vi "Set Default Config.vi"(8 "error in (no error)":errorcluster, 11 "reference in":refnum<k24>) -> (0 "error out":errorcluster, 3 "reference out":refnum<k24>)   [LabVIEW 2019, in "LabNation Scope Driver.lvlib"]
doc: "Configures the Smart Scope with default settings during start up."
uses:
  LabNation Scope Driver.lvlib
  C:/Program Files (x86)/LabNation/SmartScope/DeviceInterface.dll
  Program Files (x86)/LabNation/SmartScope/DeviceInterface.dll
  Typedef/AcquisitionMode.ctl
  Typedef/Coupling.ctl
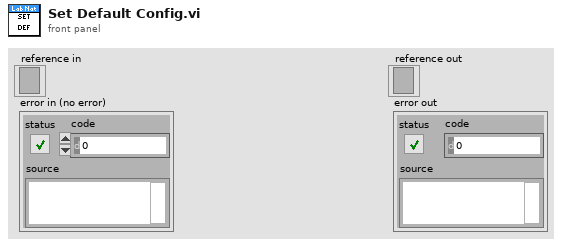
[diagram p1: front panel]
types:
  T1 = typedef "LabNation Scope Driver.lvlib/AcquisitionMode.ctl" = i32
  T2 = typedef "LabNation Scope Driver.lvlib/Coupling.ctl" = i32
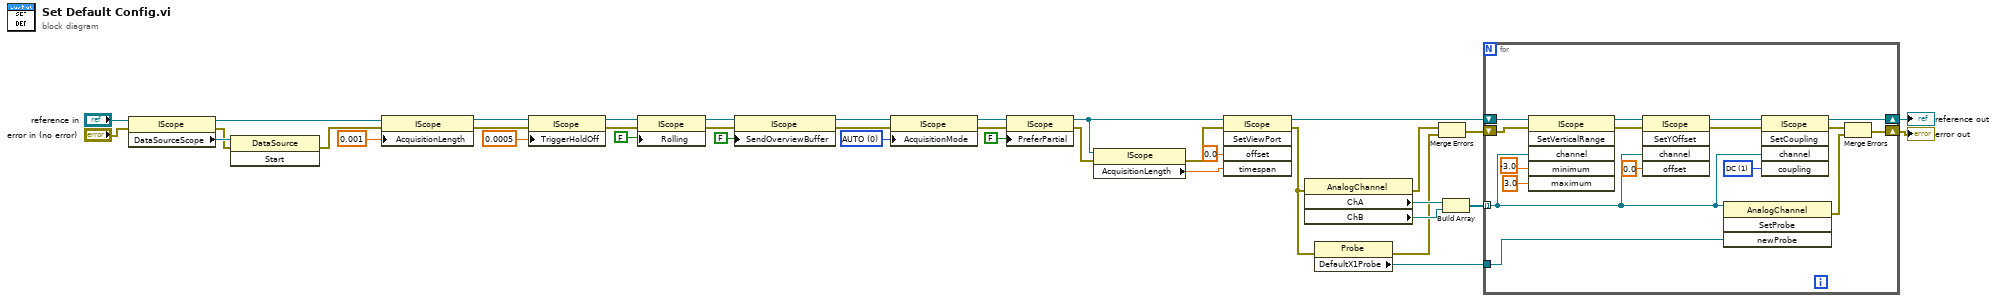
[diagram p0: block diagram]
diagram:
  w32 = T1 0 items=["AUTO", "NORMAL", "SINGLE"] ("AcquisitionMode")
  n1 = property class="IScope"(reference="reference in", error in="error in (no error)") -> (reference out=w38:refnum<k24>, error out=w18:errorcluster, "DataSourceScope"=w29:refnum<k24>)
  n2 = invoke class="DataSource" method="Start"(reference=w29, error in=w18) -> (error out=w37:errorcluster)  [unwired: 1 in, 2 out]
  n3 = property class="IScope"(reference=w38, error in=w37, "AcquisitionLength"=0.001) -> (reference out=w23:refnum<k24>, error out=w17:errorcluster)
  n4 = property class="IScope"(reference=w23, error in=w17, "TriggerHoldOff"=0.0005 ("AcquisitionLength")) -> (reference out=w24:refnum<k24>, error out=w16:errorcluster)
  n5 = property class="IScope"(reference=w24, error in=w16, "Rolling"=FALSE ("LogicAnalyserEnabled")) -> (reference out=w25:refnum<k24>, error out=w15:errorcluster)
  n6 = property class="IScope"(reference=w25, error in=w15, "SendOverviewBuffer"=FALSE) -> (reference out=w26:refnum<k24>, error out=w14:errorcluster)
  n7 = property class="IScope"(reference=w26, error in=w14, "AcquisitionMode"=w32) -> (reference out=w27:refnum<k24>, error out=w13:errorcluster)
  n8 = property class="IScope"(reference=w27, error in=w13, "PreferPartial"=FALSE) -> (reference out=w35:refnum<k24>, error out=w12:errorcluster)
  n9 = property class="IScope"(reference=w35, error in=w12) -> (error out=w11:errorcluster, "AcquisitionLength"=w36:dbl)  [unwired: 1 out]
  n10 = invoke class="IScope" method="SetViewPort"(reference=w35, error in=w11, "offset"=0.0, "timespan"=w36) -> (reference out=w20:refnum<k24>, error out=w7:errorcluster)  [unwired: 1 in, 3 out]
  n11 = property class="AnalogChannel"(error in=w7) -> (error out=w5:errorcluster, "ChA"=w19:refnum<k24>, "ChB"=w9:refnum<k24>)  [unwired: 1 in, 1 out]
  n12 = property class="Probe"(error in=w7) -> (error out=w6:errorcluster, "DefaultX1Probe"=w8:refnum<k24>)  [unwired: 1 in, 1 out]
  n13 = Merge Errors(w5, w6) -> (w4:errorcluster)
  n14 = Build Array(w19, w9) -> (w10:refnum<k24>[])
  n15 = for {
    tunnel: w10 -> [w45] mode=indexing
    shift-right: [w46] -> w3
    shift-left: w20 -> [w53]
    tunnel: w8 -> [w47]
    shift-right: [w42] -> w2
    shift-left: w4 -> [w41]
    w54 = T2 1 items=["AC", "DC"] ("coupling")
    n16 = invoke class="IScope" method="SetVerticalRange"(reference=w53, error in=w41, "channel"=w45, "minimum"=sgl -3.0, "maximum"=sgl 3.0) -> (reference out=w50:refnum<k24>, error out=w40:errorcluster)  [unwired: 1 in, 4 out]
    n17 = invoke class="IScope" method="SetYOffset"(reference=w50, error in=w40, "channel"=w45, "offset"=sgl 0.0) -> (reference out=w48:refnum<k24>, error out=w39:errorcluster)  [unwired: 1 in, 3 out]
    n18 = invoke class="AnalogChannel" method="SetProbe"(reference=w45, "newProbe"=w47) -> (error out=w43:errorcluster)  [unwired: 2 in, 3 out]
    n19 = invoke class="IScope" method="SetCoupling"(reference=w48, error in=w39, "channel"=w45, "coupling"=w54) -> (reference out=w46:refnum<k24>, error out=w44:errorcluster)  [unwired: 1 in, 3 out]
    n20 = Merge Errors(w44, w43) -> (w42:errorcluster)
  }
  "reference out" <- w3
  "error out" <- w2
